vi "4.7.vi"() -> ()   [LabVIEW 2017]
panel:
  out "猜测次数值":dbl
  out "随机的数":dbl
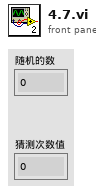
[diagram p1: front panel]
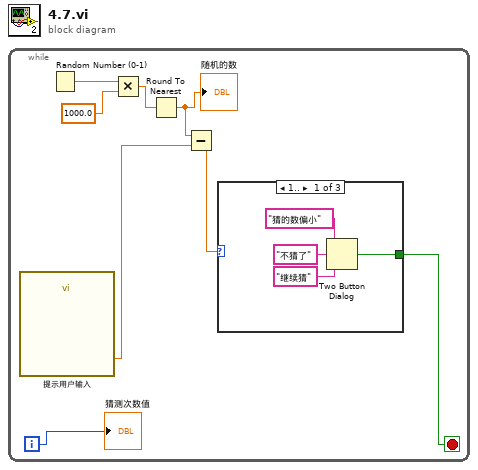
[diagram p0: block diagram]
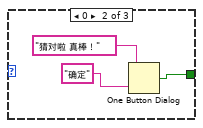
[diagram p2: hidden frame]
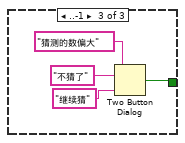
[diagram p3: hidden frame]
diagram:
  n1 = while {
    i -> [w6]
    stop <- w5 stop-if-true
    n2 = call "提示用户输入"() -> ("请在1-1000猜"=w3:dbl)  [unwired: 17 in, 2 out]
    n3 = Random Number (0-1)() -> (number: 0 to 1=w7:dbl)
    n4 = Multiply(x=w7, y=1000.0) -> (x*y=w2:dbl)
    n5 = Round To Nearest(number=w2) -> (nearest integer value=w1:dbl)
    "随机的数" <- w1
    n6 = Subtract(x=w1, y=w3) -> (x-y=w4:dbl)
    n7 = case shown="1.." w4 {
      tunnel: [w9 w13 w17] -> w5
      frame 1.. {
        n8 = Two Button Dialog(message="猜的数偏小" ("消息"), 1:"继续猜" ("F按钮名称（“取消”）"), 2:"不猜了" ("T按钮名称（“确定”）")) -> (T button?=w9:bool)
      }
      frame 0 {
        n9 = One Button Dialog(message="猜对啦 真棒！" ("消息"), button name ("OK")="确定" ("T按钮名称（“确定”）")) -> (true=w13:bool)
      }
      frame ..-1 {
        n10 = Two Button Dialog(message="猜测的数偏大" ("消息"), 1:"继续猜" ("F按钮名称（“取消”）"), 2:"不猜了" ("T按钮名称（“确定”）")) -> (T button?=w17:bool)
      }
    }
    "猜测次数值" <- w6
  }
